vi "WFS Flip 2D Array.vi"(8 "error in (no error)":errorcluster {"code" format="%.0x"}, 10 "Array YX":u32, 11 "instrument handle":refnum<visa-resource-name>) -> (0 "error out":errorcluster {"code" format="%.0x"}, 2 "Array XY":u32, 3 "instrument handle out":refnum<visa-resource-name>)   [LabVIEW 2020]
doc: "This VI flips a 2-dimensional array of size ArrayYX[MAX_SPOTS_Y (80) ][MAX_SPOTS_X (80) ] into another array ArrayXY[MAX_SPOTS_X][MAX_SPOTS_Y] with fliped x,y index order.\n\nThis VI is helpful to convert data arrays calculated by this WFS driver into a format accepted by graphic tools for display."
uses:
  WFS_32.dll
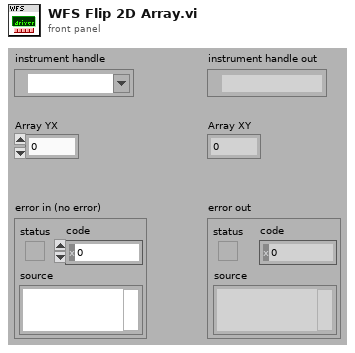
[diagram p1: front panel]
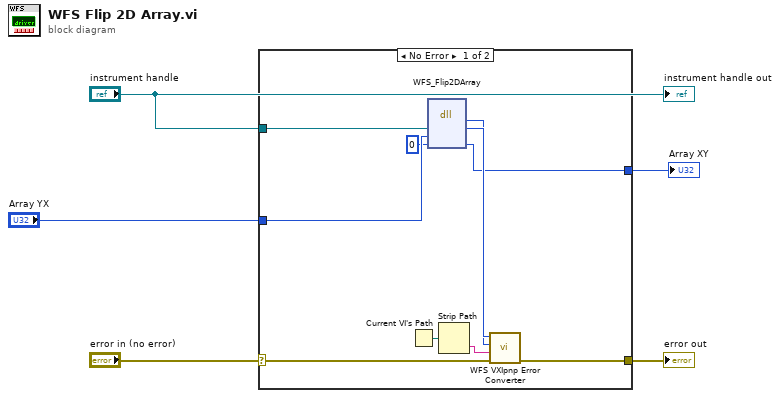
[diagram p0: block diagram]
diagram:
  n1 = case shown="No Error" "error in (no error)" {
    selector: "error in (no error)" -> [w10 w16]
    tunnel: [w9 w16] -> w5
    tunnel: "instrument handle" -> [w14 _]
    tunnel: "Array YX" -> [w8 _]
    tunnel: [w6 _] -> w1
    frame No Error {
      n2 = Current VI's Path() -> (path=w15:path)
      n3 = dll-call lib="WFS_*.*" fn="WFS_Flip2DArray"("Instrument Handle"=w14, "Array YX"=w8, "Array XY"=u32 0) -> (w12:i32, "Instrument Handle"=w13:u32, "Array XY"=w6:u32)  [unwired: 4 in, 2 out]
      n4 = Strip Path(path=w15) -> (name=w11:string)  [unwired: 1 out]
      n5 = call "WFS VXIpnp Error Converter.vi"("error in (no error)"=w10, "Name Of VI (\"\")"=w11, "CVI Error Code (0)"=w12, "instrument handle"=w13) -> ("error out"=w9:errorcluster)  [unwired: 6 in, 1 out]
    }
    frame Error {
    }
  }
  "error out" <- w5
  "Array XY" <- w1
  "instrument handle out" <- "instrument handle"
